vi "SubVI_Story.vi"() -> ()   [LabVIEW 2014]
panel:
  in  "Enter":bool
  # "在世界創始之初，宇宙共分為五大神族。於是，在經過了百億年的相互掠奪與戰爭\n過後，各族之間訂定了宇宙和平契約，並將供奉在各神殿中維持世界秩序的神殿蠟\n燭 ── 殿燭，交由契約之神代為塵封與管理，使世界維持著巧妙的平衡……。\n\n時至今日，在契約之神躺在沙發上，看他畢生中最愛的電影 ── 奇墨舅舅我 的時候\n，突然想去泡個咖啡，於是他一個轉身，就在冰箱旁磨起了咖啡豆。殊不知他家裡\n養著宇宙中最兇悍的昆蟲兼寵物 ── 強Bee 此時剛好對咖啡豆過敏，一時之間橫衝\n直撞。而在契約之神撞到強Bee之後，竟然又撞上了殿燭 的封印！！\n\n勇士們！現在是時候展現真正的技術了！拿出你們的反應與智慧，填上殿燭 中顏色\n所對應的五行密碼，在時限之內一起拯救這個世界與契約之神的飯碗吧！！"
  # "『尬電！阻止這場災難吧！』"
  # "── 契約之神 2021"
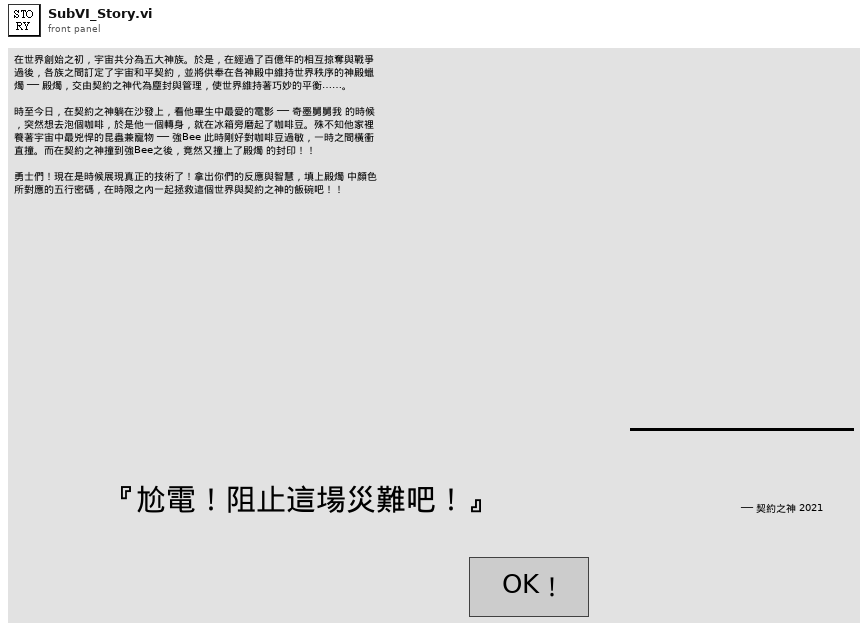
[diagram p1: front panel]
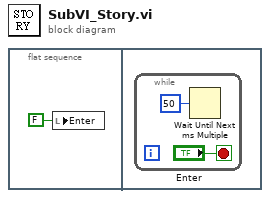
[diagram p0: block diagram]
diagram:
  n1 = flat-sequence {
    frame #0 {
      n2 = local write "Enter"(FALSE ("Enter")) -> ()
    }
    frame #1 {
      n3 = while {
        stop <- "Enter" stop-if-true
        n4 = Wait Until Next ms Multiple(millisecond multiple=u32 50 ("milliseconds to wait")) -> ()  [unwired: 1 out]
      }
    }
  }
